vi "CRYGet Line Infor.vi"(0 "This VI":refnum<vi>, 1 "Active Plot Number":u16, 2 "Graph Type":string="LineStyle", 3 "XY Graph Control Ref":refnum<vi>, 4 "Wave Graph Control Ref":refnum<vi>, 8 "Property Set?":bool) -> (14 "Line":u32(colorbox), 16 "Point/Fill":u32(colorbox), 18 "Fill to":i16(ring) items=["<none>"=-1, "zero"=-2, "-Infinity"=-3, "+Infinity"=-4], 20 "LineStyle":string, 21 "LineWidth":string, 22 "PointStyle":string, 23 "Interpolation":string)   [LabVIEW 2013]
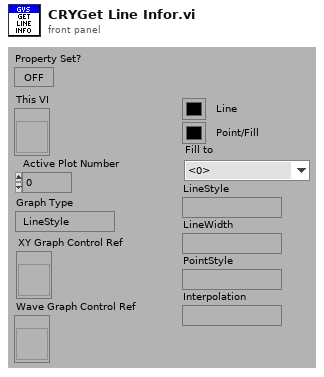
[diagram p1: front panel]
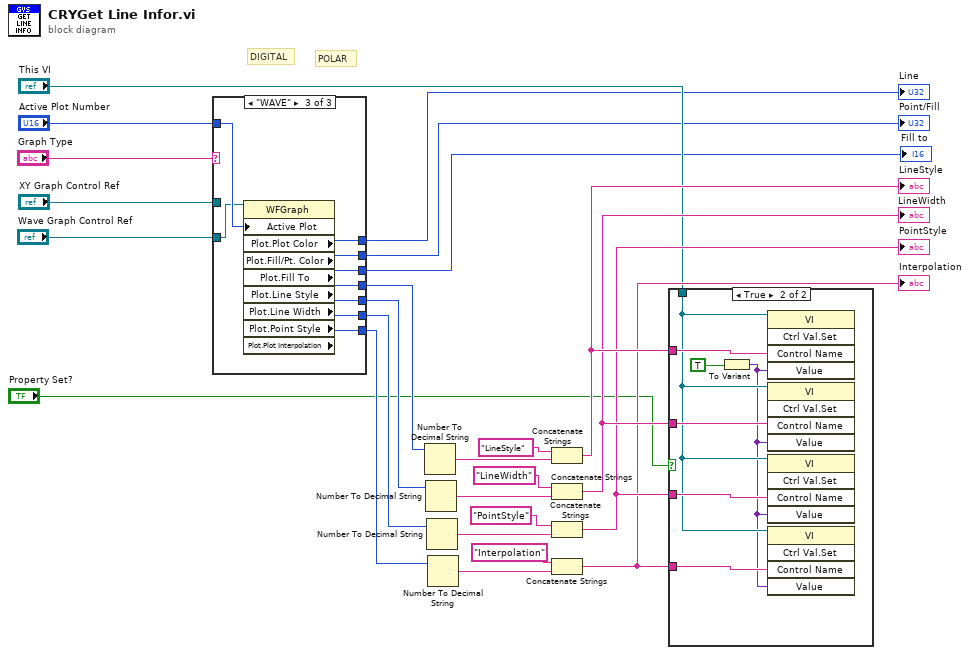
[diagram p0: block diagram]
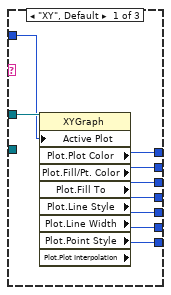
[diagram p3: hidden frame]
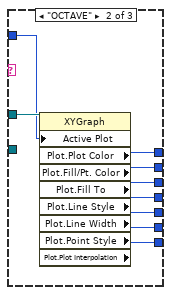
[diagram p4: hidden frame]
diagram:
  # "POLAR"
  # "DIGITAL"
  n1 = case shown="\"WAVE\"" "Graph Type" {
    tunnel: "XY Graph Control Ref" -> [w34 w43 _]
    tunnel: "Active Plot Number" -> [w33 w42 w52]
    tunnel: [w32 w41 w51] -> w10
    tunnel: [w31 w40 w50] -> w9
    tunnel: [w30 w39 w49] -> w8
    tunnel: [w29 w38 w48] -> w7
    tunnel: [w28 w37 w47] -> w6
    tunnel: [w27 w36 w46] -> w5
    tunnel: [w26 w35 w45] -> w4
    tunnel: "Wave Graph Control Ref" -> [_ _ w44]
    frame "XY", Default {
      n2 = property class="XYGraph"(reference=w34, "Active Plot"=w33) -> ("Plot.Plot Color"=w32:u32, "Plot.Fill/Pt. Color"=w31:u32, "Plot.Fill To"=w30:i16, "Plot.Line Style"=w29:u8, "Plot.Line Width"=w28:u8, "Plot.Point Style"=w27:u8, "Plot.Plot Interpolation"=w26:u8)  [unwired: 1 in, 2 out]
    }
    frame "OCTAVE" {
      n3 = property class="XYGraph"(reference=w43, "Active Plot"=w42) -> ("Plot.Plot Color"=w41:u32, "Plot.Fill/Pt. Color"=w40:u32, "Plot.Fill To"=w39:i16, "Plot.Line Style"=w38:u8, "Plot.Line Width"=w37:u8, "Plot.Point Style"=w36:u8, "Plot.Plot Interpolation"=w35:u8)  [unwired: 1 in, 2 out]
    }
    frame "WAVE" {
      n4 = property class="WFGraph"(reference=w44, "Active Plot"=w52) -> ("Plot.Plot Color"=w51:u32, "Plot.Fill/Pt. Color"=w50:u32, "Plot.Fill To"=w49:i16, "Plot.Line Style"=w48:u8, "Plot.Line Width"=w47:u8, "Plot.Point Style"=w46:u8, "Plot.Plot Interpolation"=w45:u8)  [unwired: 1 in, 2 out]
    }
  }
  "Line" <- w10
  "Point/Fill" <- w9
  "Fill to" <- w8
  n5 = Number To Decimal String(number=w7) -> (decimal integer string=w25:string)  [unwired: 1 out]
  n6 = Number To Decimal String(number=w6) -> (decimal integer string=w24:string)  [unwired: 1 out]
  n7 = Number To Decimal String(number=w5) -> (decimal integer string=w23:string)  [unwired: 1 out]
  n8 = Number To Decimal String(number=w4) -> (decimal integer string=w22:string)  [unwired: 1 out]
  n9 = Concatenate Strings("LineStyle", w25) -> (w17:string)
  "LineStyle" <- w17
  n10 = Concatenate Strings("LineWidth", w24) -> (w16:string)
  "LineWidth" <- w16
  n11 = Concatenate Strings("PointStyle", w23) -> (w15:string)
  "PointStyle" <- w15
  n12 = Concatenate Strings("Interpolation", w22) -> (w14:string)
  "Interpolation" <- w14
  n13 = case shown="True" "Property Set?" {
    tunnel: w17 -> [_ w59]
    tunnel: w16 -> [_ w58]
    tunnel: w15 -> [_ w57]
    tunnel: w14 -> [_ w56]
    tunnel: "This VI" -> [_ w55]
    frame False {
    }
    frame True {
      n14 = To Variant(anything=TRUE) -> (Variant=w53:variant)
      n15 = invoke class="VI" method="Ctrl Val.Set"(reference=w55, "Control Name"=w59, "Value"=w53) -> ()  [unwired: 2 in, 5 out]
      n16 = invoke class="VI" method="Ctrl Val.Set"(reference=w55, "Control Name"=w58, "Value"=w53) -> ()  [unwired: 2 in, 5 out]
      n17 = invoke class="VI" method="Ctrl Val.Set"(reference=w55, "Control Name"=w57, "Value"=w53) -> ()  [unwired: 2 in, 5 out]
      n18 = invoke class="VI" method="Ctrl Val.Set"(reference=w55, "Control Name"=w56, "Value"=w53) -> ()  [unwired: 2 in, 5 out]
    }
  }
